vi "Validation.vi"(9 "Date":string="2018111317", 11 "Password":string) -> (0 "激活状态":i32, 2 "ComputureID":string, 3 "提示符":string)   [LabVIEW 2018]
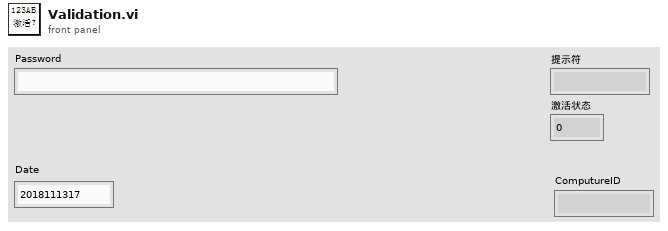
[diagram p1: front panel]
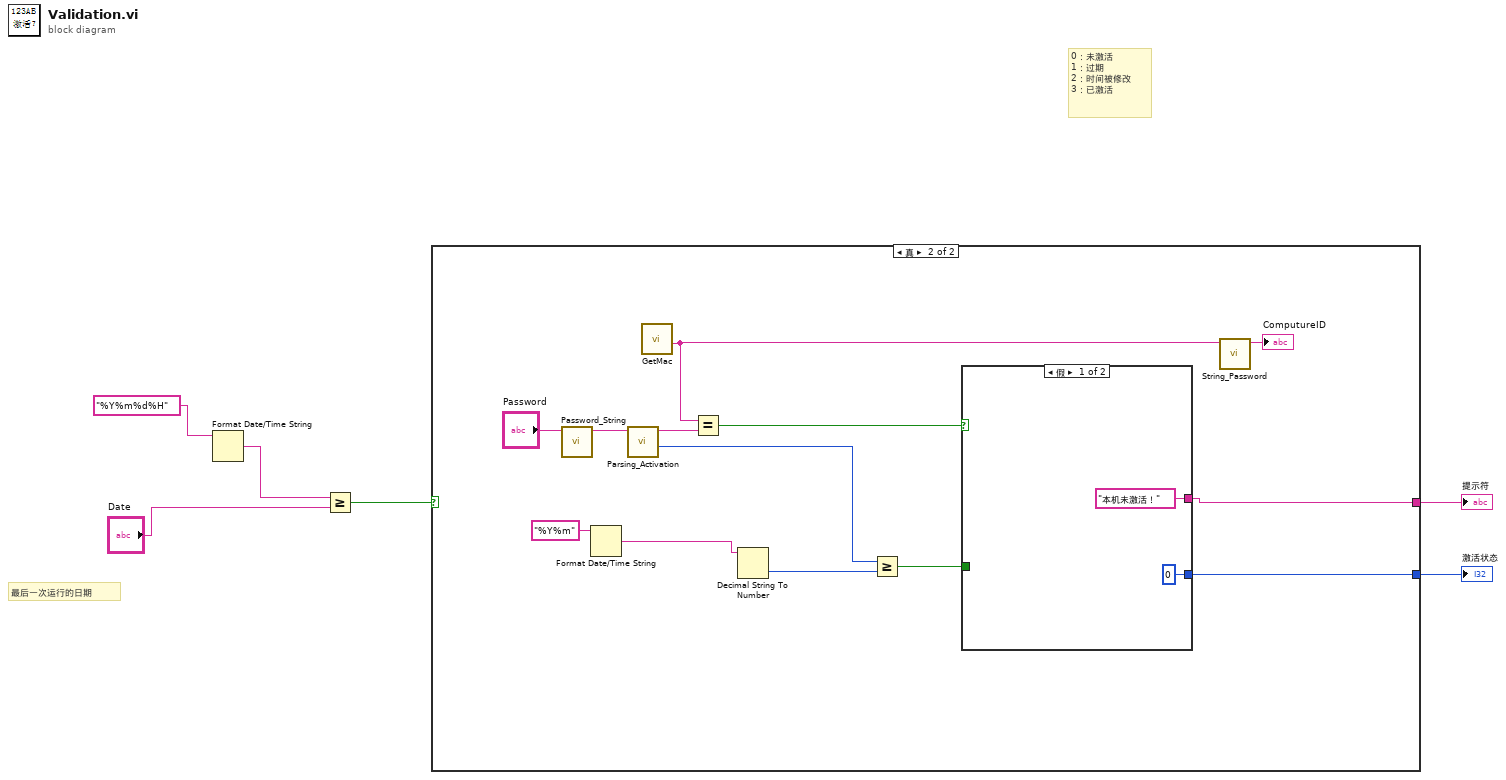
[diagram p0: block diagram]
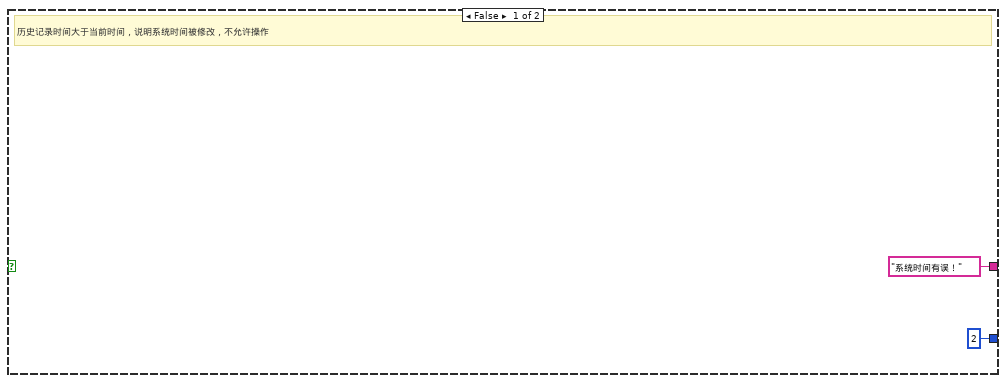
[diagram p2: hidden frame]
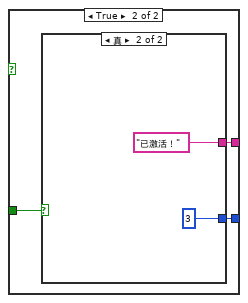
[diagram p3: hidden frame]
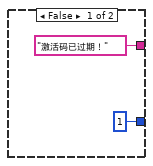
[diagram p4: hidden frame]
diagram:
  # "0：未激活\n1：过期\n2：时间被修改\n3：已激活"
  # "最后一次运行的日期"
  n1 = Format Date/Time String(time format string (%c)="%Y%m%d%H" ("时间格式字符串(%c)")) -> (date/time string=w1:string)  [unwired: 2 in]
  n2 = Greater Or Equal?(x=w1, y="Date") -> (x >= y?=w4:bool)
  n3 = case shown="真" w4 {
    tunnel: ["系统时间有误！" w11] -> w6
    tunnel: [2 w10] -> w5
    frame False {
      # "历史记录时间大于当前时间，说明系统时间被修改，不允许操作"
    }
    frame True {
      n4 = call "Password_String.vi"("Password"="Password") -> ("String"=w19:string)  [unwired: 10 in]
      n5 = Format Date/Time String(time format string (%c)="%Y%m" ("时间格式字符串(%c)")) -> (date/time string=w9:string)  [unwired: 2 in]
      n6 = call "Parsing_Activation.vi"("ActivationCode"=w19) -> ("使用期限"=w17:i32, "MAC"=w18:string)  [unwired: 9 in]
      n7 = call "GetMac.vi"() -> ("网络适配器:MAC地址"=w14:string)  [unwired: 10 in, 1 out]
      n8 = Equal?(x=w14, y=w18) -> (x = y?=w15:bool)
      n9 = Decimal String To Number(string=w9) -> (number=w16:i32)  [unwired: 2 in, 1 out]
      n10 = Greater Or Equal?(x=w17, y=w16) -> (x >= y?=w12:bool)
      n11 = case shown="假" w15 {
        tunnel: ["本机未激活！" w26] -> w11
        tunnel: [0 w25] -> w10
        tunnel: w12 -> [_ w24]
        frame False {
        }
        frame True {
          n12 = case shown="真" w24 {
            tunnel: ["激活码已过期！" "已激活！"] -> w26
            tunnel: [1 3] -> w25
            frame False {
            }
            frame True {
            }
          }
        }
      }
      n13 = call "String_Password.vi"("String"=w14) -> ("Password"=→"ComputureID":string)  [unwired: 10 in]
    }
  }
  "提示符" <- w6
  "激活状态" <- w5
